vi "mult_CFO_sync_single.vi"(8 "CP length":u32=64, 9 "FFT size":u32=256, 11 "time samples":cdb[](array[numeric])) -> (3 "sync ofdm symbol":cdb[](array[numeric]))   [LabVIEW 2020]
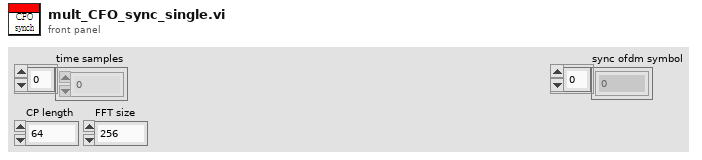
[diagram p1: front panel]
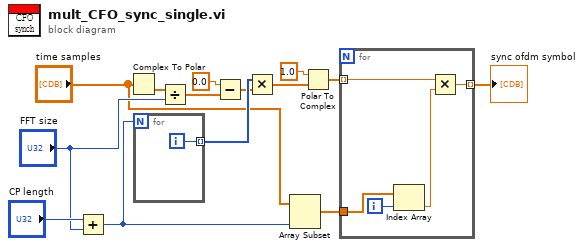
[diagram p0: block diagram]
diagram:
  n1 = Add(x="CP length", y="FFT size") -> (x+y=w12:u32)
  n2 = Complex To Polar(r * e^(i*theta)="time samples") -> (theta=w14:dbl[])  [unwired: 1 out]
  n3 = for {
    N: w12 -> [_]
    tunnel: [w15] -> w10 mode=indexing
    i -> [w15]
  }
  n4 = Divide(x=w14, y="FFT size") -> (x/y=w6:dbl[])
  n5 = Subtract(x=0.0, y=w6) -> (x-y=w9:dbl[])
  n6 = Multiply(x=w10, y=w9) -> (x*y=w8:dbl[])
  n7 = Array Subset(array="time samples", length=w12) -> (w5:cdb[])  [unwired: 1 in]
  n8 = Polar To Complex(1:w8, 2:1.0) -> (0:w7:cdb[])
  n9 = for {
    tunnel: w7 -> [w17] mode=indexing
    tunnel: w5 -> [w20]
    tunnel: [w16] -> w4 mode=indexing
    i -> [w19]
    n10 = Index Array(array=w20, index=w19) -> (element=w18:cdb)
    n11 = Multiply(x=w17, y=w18) -> (x*y=w16:cdb)
  }
  "sync ofdm symbol" <- w4
